vi "ConfigDevice.vi"(0 "Device in":refnum<class "Device.lvclass">, 12 "ConfigInterface":refnum<class "ConfigInterface.lvclass">, 13 "MessageInterface":refnum<class "MessageInterface.lvclass">, 14 "SV_Publisher":refnum<class "SV_Publisher.lvclass">) -> (4 "Device out":refnum<class "Device.lvclass">)   [LabVIEW 2019, in "Device.lvclass"]
uses:
  Device.lvclass
  MessageInterface_class/MessageInterface.lvclass
  ConfigInterface_class/ConfigInterface.lvclass
  SV_Puplisher_class/SV_Publisher.lvclass
  Device.lvclass/Device.ctl
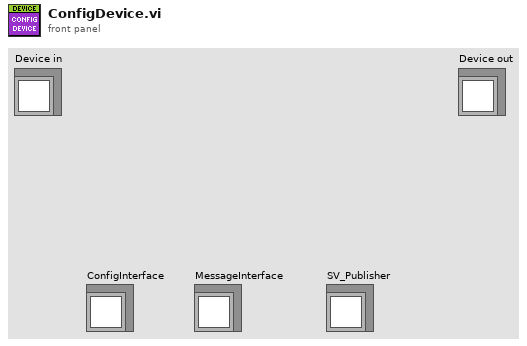
[diagram p1: front panel]
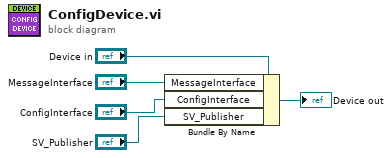
[diagram p0: block diagram]
diagram:
  n1 = Bundle By Name(cluster="Device in", "MessageInterface"="MessageInterface", "ConfigInterface"="ConfigInterface", "SV_Publisher"="SV_Publisher") -> (→"Device out":refnum<class "Device.lvclass">)
